vi "SSC Digital Fetch Capture Waveform.vi"(0 "Digital SSC in":T1[](array[typedef]), 1 "Waveform Name":string, 7 "timeout (s)":dbl=10.0, 9 "samples to read":i32, 11 "error in":errorcluster) -> (4 "Digital SSC out":T1[](array[typedef]), 6 "Per-Instrument Capture":u32[][][](array[numeric]), 15 "error out":errorcluster)   [LabVIEW 2020]
doc: "Fetches a defined number of samples for the sites connected to the specified pin(s) and pin group(s). This VI only returns data from sites that are enabled when fetch is called."
uses:
  SSC Digital.ctl
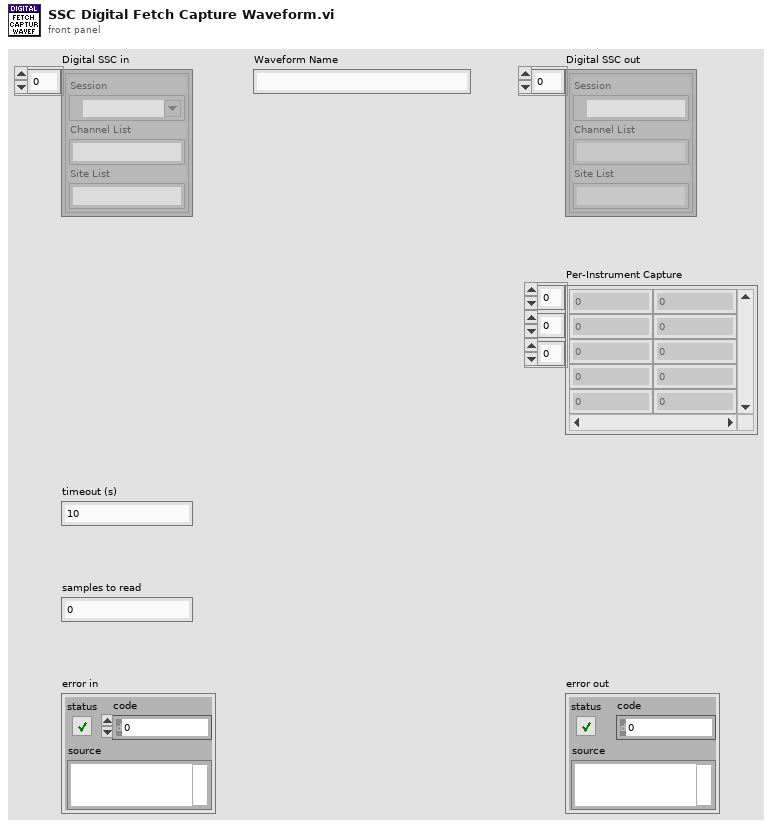
[diagram p1: front panel]
types:
  T1 = typedef "SSC Digital.ctl" = cluster{"Session":refnum<k15>, "Channel List":string, "Site List":string}
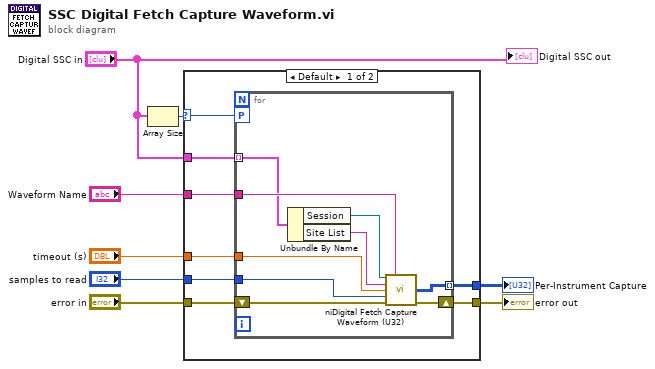
[diagram p0: block diagram]
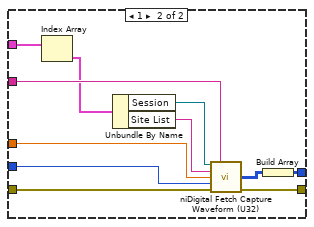
[diagram p2: hidden frame]
diagram:
  n1 = Array Size(array="Digital SSC in") -> (size(s)=w2:i32)
  n2 = case shown="Default" w2 {
    selector: w2 -> [w10 _]
    tunnel: "Waveform Name" -> [w16 w36]
    tunnel: "timeout (s)" -> [w15 w35]
    tunnel: "samples to read" -> [w14 w34]
    tunnel: "error in" -> [w13 w33]
    tunnel: [w12 w32] -> w4
    tunnel: [w11 w26] -> w3
    tunnel: "Digital SSC in" -> [w9 w30]
    frame Default {
      n3 = for {
        tunnel: w16 -> [w25]
        workers-P: w10 -> [_]
        tunnel: [w20] -> w11 mode=indexing
        tunnel: w15 -> [w22]
        tunnel: w14 -> [w21]
        shift-right: [w23] -> w12
        shift-left: w13 -> [w24]
        tunnel: w9 -> [w19] mode=indexing
        n4 = Unbundle By Name(w19) -> ("Session"=w18:refnum<k15>, "Site List"=w17:string)
        n5 = call <instrlib>:"niDigital Fetch Capture Waveform (U32).vi"("instrument handle"=w18, "waveform name"=w25, "site list"=w17, "timeout (s)"=w22, "samples to read"=w21, "error in"=w24) -> ("data"=w20:u32[][], "error out"=w23:errorcluster)  [unwired: 7 in, 1 out]
      }
    }
    frame 1 {
      n6 = Index Array(array=w30) -> (element=w27:T1)  [unwired: 1 in]
      n7 = Unbundle By Name(w27) -> ("Session"=w29:refnum<k15>, "Site List"=w28:string)
      n8 = call <instrlib>:"niDigital Fetch Capture Waveform (U32).vi"("instrument handle"=w29, "waveform name"=w36, "site list"=w28, "timeout (s)"=w35, "samples to read"=w34, "error in"=w33) -> ("data"=w31:u32[][], "error out"=w32:errorcluster)  [unwired: 7 in, 1 out]
      n9 = Build Array(w31) -> (w26:u32[][][])
    }
  }
  "error out" <- w4
  "Per-Instrument Capture" <- w3
  "Digital SSC out" <- "Digital SSC in"
